vi "BooleanToStr(cast).vi"(1 "布尔":bool) -> (0 "字符串":string)   [LabVIEW 2012]
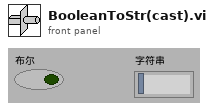
[diagram p1: front panel]
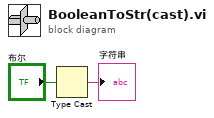
[diagram p0: block diagram]
diagram:
  n1 = Type Cast(x="布尔") -> (*(type *) &x=→"字符串":string)  [unwired: 1 in]
